vi "stop_condition_i2c.vi"   [LabVIEW 2019]
uses:
  <vilib>/rvi/eio/common/nirviEmuTemplateMethod_errors.vi
  <vilib>/eio/EIONode/EIONode.xnode
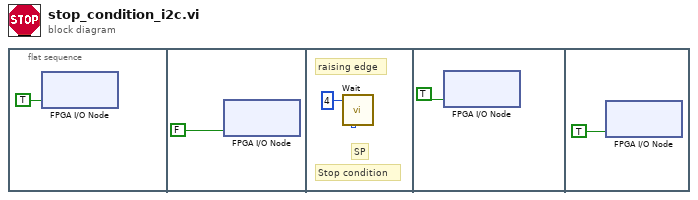
[diagram p0: block diagram]
diagram:
  n1 = flat-sequence {
    frame #0 {
      n2 = xnode "FPGA I/O Node"("SCL"=TRUE) -> ()  [unwired: 1 in, 1 out]
    }
    frame #1 {
      n3 = xnode "FPGA I/O Node"("SDA"=FALSE) -> ()  [unwired: 1 in, 1 out]
    }
    frame #2 {
      # "SP"
      # "Stop condition"
      # "raising edge"
      n4 = call "Wait"("Count(Ticks)"=u32 4) -> ()  [unwired: 1 out]
    }
    frame #3 {
      n5 = xnode "FPGA I/O Node"("SCL"=TRUE) -> ()  [unwired: 1 in, 1 out]
    }
    frame #4 {
      n6 = xnode "FPGA I/O Node"("SDA"=TRUE) -> ()  [unwired: 1 in, 1 out]
    }
  }
